vi "指定范围的随机数2D(dbl).vi"(6 "下限 (0.00)":dbl format="%.2f", 7 "上限 (1.00)":dbl=1.0 format="%.2f", 8 "Error In":errorcluster caption="错误输入", 9 "Clol":i32, 10 "Row":i32) -> (0 "Error Out":errorcluster caption="错误输出", 3 "随机数":dbl[][](array[numeric]))   [LabVIEW 2013]
doc: "功能：\n\n产生指定范围的<b>随机数</b>。\n\n\n\n\n\ncsxcs_366创建"
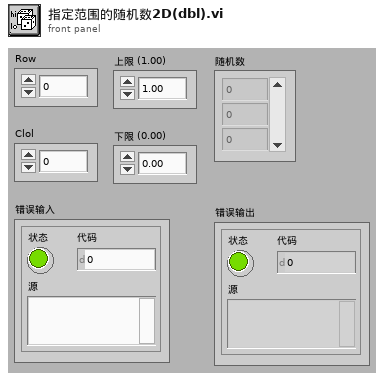
[diagram p1: front panel]
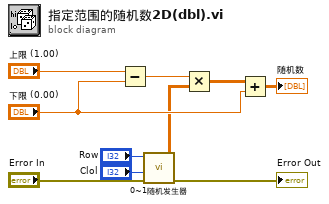
[diagram p0: block diagram]
diagram:
  n1 = Subtract(x="上限 (1.00)", y="下限 (0.00)") -> (x-y=w8:dbl)
  n2 = call-poly "0~1随机发生器.vi"("Error In"="Error In", "Clol"="Clol", "Row"="Row") -> ("Error Out"=→"Error Out":errorcluster, "Rand(0~1) 2D"=w5:dbl[][])  [unwired: 7 in]
  n3 = Multiply(x=w8, y=w5) -> (x*y=w6:dbl[][])
  n4 = Add(x=w6, y="下限 (0.00)") -> (x+y=→"随机数":dbl[][])
